vi "Quadrature Encoder dX Method (FPGA, Use in SCTL).vi"(0 "Clock":bool, 1 "Reset Enc":bool, 2 "A":bool, 3 "B":bool, 4 "Z":bool, 5 "Polarity":bool, 7 "Clock Divider":u16=1, 9 "Reset Position":i32) -> (14 "Vel/Acc Update":bool, 15 "Position (Counts)":i32, 16 "Velocity (Counts/Interval)":i32, 17 "Acceleration (Counts/Interval^2)":i32, 18 "dT (Ticks)":u32, 19 "CW Direction":bool)   [LabVIEW 2014]
doc: "Calculates 32-bit position, velocity, and acceleration based on a Quadrature encoder signal. This function resets the position upon the first Z index pulse. Subsequent Z index pulses are ignored. The velocity and acceleration values are not effected when the position is reset by the Z index pulse. The Direction input determines whether the function counts up or down based on clockwise motion.\n\nOPERATION\nUses A, B, and Z index signals to calculate position. Upon the falling edge of the Clock input, the function updates the position, velocity, acceleration, and elapsed time and latches the result. The velocity is calculated in units of Counts/Interval by subtracting the current position from the previous position. The acceleration is calculated in units of Counts/Interval^2 by subtracting the current velocity from the previous velocity.\n\nThe Clock Divider signal increases the time interval between velocity and acceleration estimates by N number of clocks to provide better resolution when the time interval between clock updates is small. Since more encoder counts are acquired during the time interval, the accuracy increases. The drawback is that the time delay also increases for the velocity and acceleration updates. The position always updates on every rising clock edge. If Clock Divider is set to 0 the Clock signal is ignored and the position, velocity, and acceleration are updated each time the function is called.\n\nThis function should be run as fast as possible to ensure that no Quadrature encoder digital edges are missed. Do not add delay timers into the loop containing this function.\n\nIf the encoder signals are noise, you may want to use the Filter Digital Lines, 3-ch (FPGA).vi function on the A, B, and Z signals before feeding them into this Quadrature encoder function.\n\nRT HOST INTERFACE\nIn your RT host application, you can divide Velocity (Counts/Interval) by the time interval dT (Ticks) to convert the velocity to units of Counts/Tick. By default, one tick is equal to 25 nanoseconds (40 MHz), so you can calculate the velocity in units of Counts per Second as follows,\n\nVelocity (Counts/s) = Velocity (Counts/Interval) / [dT (Ticks) * 25e-9 (s)]\n\nIn your RT host application, you can divide Acceleration (Counts/Interval^2) by the square of the time interval (dT (Ticks))^2 to convert the acceleration to units of Counts/Tick^2. By default, one tick is equal to 25 nanoseconds (40 MHz), so you can calculate the acceleration in units of Counts per Second^2 as follows,\n\nAcceleration (Counts/s^2) = Acceleration (Counts/Interval^2) / [(dT (Ticks))^2 * 25e-9^2 (s^2)]\n\nINPUTS\nClock- Falling edge latches the position, velocity, acceleration, and elapsed time\nReset- Sets the position to the Reset Position value\nA- Quadrature encoder A phase signal\nB- Quadrature encoder B phase signal\nZ- Quadrature encoder Z index signal\nPolarity- When FALSE, counterclockwise motion causes the Position (Counts) output to increment\nClock Divider- Causes the velocity and acceleration values to update every N clocks\nReset Position- The position will be set to this value when the first Z index pulse occurs or the Reset input is asserted\nVel/Acc Update- Boolean signal that changes state when the velocity and acceleration outputs are updated. Used for synchronization with other loops.\nCW Direction- If the Polarity input is FALSE, this signal is TRUE when clockwise motion is detected\n\n\nOUTPUTS\nPosition (Counts)- The position count value, updated continuously\nVelocity (Counts/Interval)- The amount the position has changed between the last two updates\nAcceleration (Counts/Interval^2)- The amount the velocity has changed between the last two updates\ndT (Ticks)- The time interval between velocity and acceleration updates, express in FPGA clock ticks\n\nNOTES\nBy allowing more time between updates you obtain more averaging on the velocity and acceleration values and therefore smoother results. A larger time interval results in less noise on the velocity and acceleration calculations. Also, using an encoder with more counts per revolution results in better accuracy and smoother results on the velocity and acceleration calculations.\n\nSaturation Subtract functions are used to saturate the signed velocity and acceleration values in the case of integer overflow. \n\nA normal Subtract function is used on the elapsed time counter. Because unsigned integers are used, the dT (Ticks) value is correct even when the Tick Count value rolls over."
uses:
  <vilib>/rvi/Emulation/niFpgaProcessEmulError.vi
  Instance           2 56Saved   Quadrature Encoder dX Method (FPGA, Use in SCTL) .vi
  Instance           1 56Saved   Quadrature Encoder dX Method (FPGA, Use in SCTL) .vi
  <vilib>/rvi/Emulation/niFpgaSctlEmulationGetInTimedLoop.vi
  <vilib>/rvi/Arithmetic/AddSubMult/XNode/nirviSatArithmetic.xnode
panel:
  out "R9":u16
  out "R8":bool
  out "R7":u32
  out "R6":i32
  out "R5":i32
  out "R4":i32
  out "R3":bool
  out "R2":bool
  out "R1":bool
  # "Internal Registers"
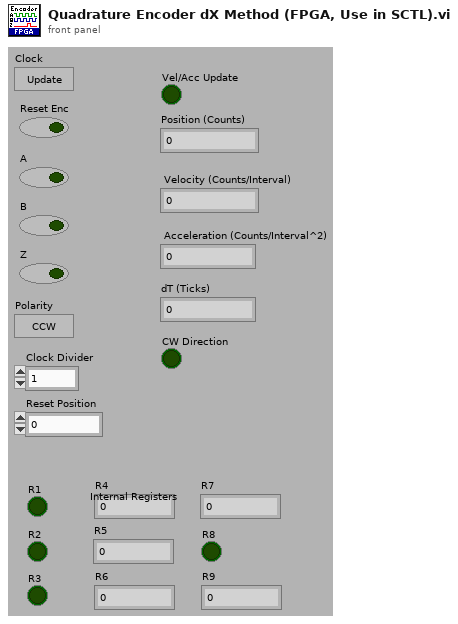
[diagram p1: front panel]
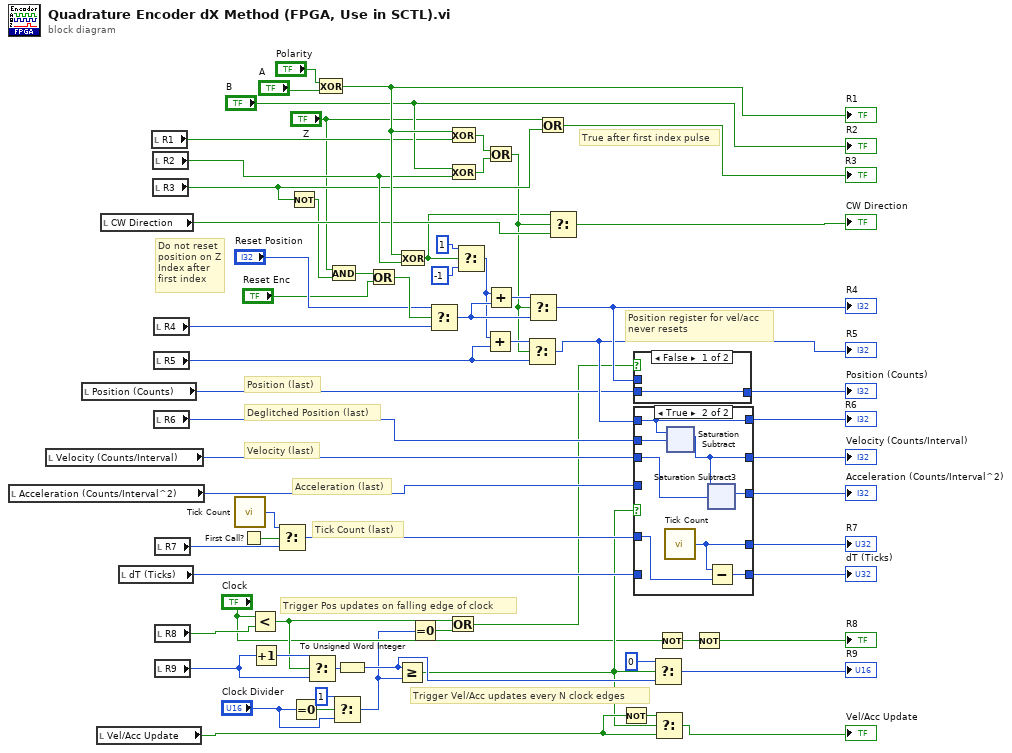
[diagram p0: block diagram]
diagram:
  # "Trigger Vel/Acc updates every N clock edges"
  # "Trigger Pos updates on falling edge of clock"
  # "Position (last)"
  # "Tick Count (last)"
  # "Position register for vel/acc\nnever resets"
  # "True after first index pulse"
  # "Acceleration (last)"
  # "Velocity (last)"
  # "Deglitched Position (last)"
  # "Do not reset position on Z Index after first index"
  n1 = local read "Acceleration (Counts/Interval^2)"() -> (w42:i32)
  n2 = local read "Velocity (Counts/Interval)"() -> (w43:i32)
  n3 = local read "Position (Counts)"() -> (w45:i32)
  n4 = local read "Vel/Acc Update"() -> (w37:bool)
  n5 = local read "CW Direction"() -> (w48:bool)
  n6 = local read "dT (Ticks)"() -> (w40:u32)
  n7 = local read "R1"() -> (w51:bool)
  n8 = local read "R2"() -> (w50:bool)
  n9 = local read "R3"() -> (w49:bool)
  n10 = local read "R4"() -> (w47:i32)
  n11 = local read "R5"() -> (w46:i32)
  n12 = local read "R6"() -> (w44:i32)
  n13 = local read "R7"() -> (w41:u32)
  n14 = local read "R8"() -> (w39:bool)
  n15 = local read "R9"() -> (w38:u16)
  n16 = call "Tick Count"() -> ("Tick Count(Ticks)"=w7:u32)
  n17 = First Call?() -> (First Call?: T/F=w29:bool)
  n18 = Less?(x="Clock", y=w39) -> (x < y?=w25:bool)
  n19 = Increment(x=w38) -> (x+1=w27:u16)
  n20 = Select(t=w7, s=w29, f=w41) -> (s? t:f=w28:u32)
  n21 = Not(x=w49) -> (.not. x?=w30:bool)
  n22 = Equal To 0?(x="Clock Divider") -> (x = 0?=w5:bool)
  n23 = Select(t=w27, s=w25, f=w38) -> (s? t:f=w26:u16)
  n24 = Exclusive Or(1:"A", 2:"Polarity") -> (0:w60:bool)
  "R1" <- w60
  n25 = And(x="Z", y=w30) -> (x .and. y?=w20:bool)
  n26 = Select(t=u16 1, s=w5, f="Clock Divider") -> (s? t:f=w2:u16)
  n27 = To Unsigned Word Integer(number=w26) -> (unsigned 16bit integer=w24:u16)
  n28 = Or(x=w20, y="Reset Enc") -> (x .or. y?=w19:bool)
  n29 = Greater Or Equal?(x=w24, y=w2) -> (x >= y?=w15:bool)
  n30 = Exclusive Or(1:w50, 2:w60) -> (0:w12:bool)
  n31 = Equal To 0?(x=w2) -> (x = 0?=w21:bool)
  n32 = Select(t="Reset Position", s=w19, f=w47) -> (s? t:f=w35:i32)
  n33 = Or(x=w25, y=w21) -> (x .or. y?=w22:bool)
  n34 = Exclusive Or(1:w51, 2:w60) -> (0:w31:bool)
  n35 = Exclusive Or(1:w50, 2:"B") -> (0:w32:bool)
  n36 = Select(t=1 ("32 bit"), s=w12, f=-1 ("32 bit")) -> (s? t:f=w17:i32)
  n37 = Add(x=w17, y=w46) -> (x+y=w18:i32)
  n38 = Or(x=w31, y=w32) -> (x .or. y?=w13:bool)
  n39 = Add(x=w17, y=w35) -> (x+y=w36:i32)
  n40 = Select(t=w18, s=w13, f=w46) -> (s? t:f=w56:i32)
  "R5" <- w56
  n41 = Select(t=w36, s=w13, f=w35) -> (s? t:f=w57:i32)
  "R4" <- w57
  n42 = Or(x="Z", y=w49) -> (x .or. y?=→"R3":bool)
  n43 = Select(t=w12, s=w13, f=w48) -> (s? t:f=→"CW Direction":bool)
  n44 = Not(x=w37) -> (.not. x?=w16:bool)
  n45 = case shown="False" w22 {
    tunnel: w57 -> [_ w68]
    tunnel: w45 -> [w67 _]
    tunnel: [w67 w68] -> w66
    frame False {
    }
    frame True {
    }
  }
  "Position (Counts)" <- w66
  n46 = case shown="True" w15 {
    tunnel: w56 -> [_ w81]
    tunnel: [w73 w81] -> w55
    tunnel: w44 -> [w73 w80]
    tunnel: [w72 w79] -> w65
    tunnel: w43 -> [w72 w78]
    tunnel: [w71 w77] -> w64
    tunnel: w42 -> [w71 _]
    tunnel: [w70 w76] -> w63
    tunnel: w40 -> [w70 _]
    tunnel: [w69 w75] -> w54
    tunnel: w28 -> [w69 w74]
    frame False {
    }
    frame True {
      n47 = call "Tick Count"() -> ("Tick Count(Ticks)"=w75:u32)
      n48 = xnode ("Saturation Subtract")("x"=w81, "y"=w80) -> ("x-y"=w79:i32)
      n49 = Subtract(x=w75, y=w74) -> (x-y=w76:u32)
      n50 = xnode ("Saturation Subtract3")("x"=w79, "y"=w78) -> ("x-y"=w77:i32)
    }
  }
  "Velocity (Counts/Interval)" <- w65
  "Acceleration (Counts/Interval^2)" <- w64
  "dT (Ticks)" <- w63
  "R6" <- w55
  "R7" <- w54
  n51 = Select(t=u16 0, s=w15, f=w24) -> (s? t:f=→"R9":u16)
  n52 = Select(t=w16, s=w15, f=w37) -> (s? t:f=→"Vel/Acc Update":bool)
  n53 = Not(x="Clock") -> (.not. x?=w1:bool)
  n54 = Not(x=w1) -> (.not. x?=→"R8":bool)
  "R2" <- "B"
